vi "Power Enabled.vi"(0 "P CH":refnum<vi>, 1 "P CH_char":refnum<vi>, 2 "P CH, V":refnum<vi>, 3 "P CH_curlim, A":refnum<vi>, 4 "P CH_cur, A":refnum<vi>, 5 "P CH_selcur, A":refnum<vi>, 6 "P CH_counter":refnum<vi>, 7 "P CH_warning":refnum<vi>, 10 "P CH Used":bool, 16 "Stop":bool) -> ()   [LabVIEW 2018]
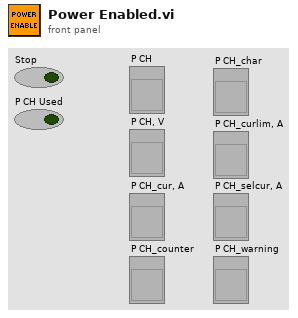
[diagram p1: front panel]
types:
  T1 = enum8{"Enabled", "Disabled", "Disabled and Grayed Out"}
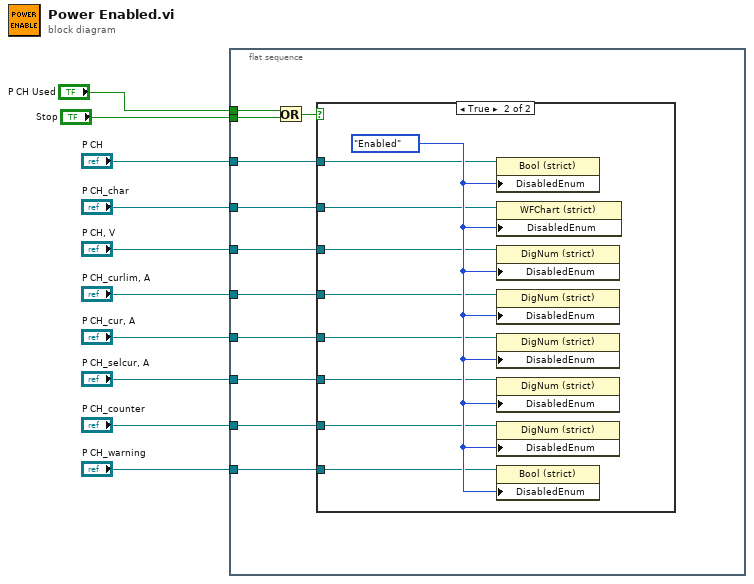
[diagram p0: block diagram]
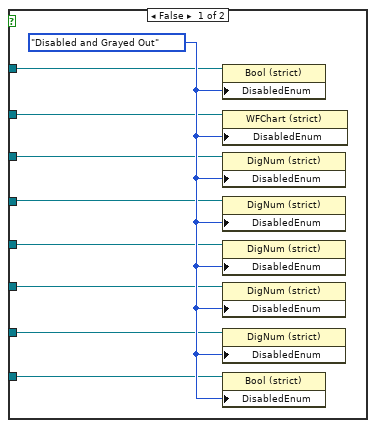
[diagram p2: hidden frame]
diagram:
  n1 = flat-sequence {
    tunnel: "Stop" -> [w20]
    tunnel: "P CH Used" -> [w19]
    tunnel: "P CH" -> [w18]
    tunnel: "P CH_char" -> [w17]
    tunnel: "P CH, V" -> [w16]
    tunnel: "P CH_curlim, A" -> [w15]
    tunnel: "P CH_cur, A" -> [w14]
    tunnel: "P CH_selcur, A" -> [w13]
    tunnel: "P CH_counter" -> [w12]
    tunnel: "P CH_warning" -> [w11]
    frame #0 {
      n2 = Or(x=w19, y=w20) -> (x .or. y?=w21:bool)
      n3 = case shown="True" w21 {
        tunnel: w18 -> [w29 w38]
        tunnel: w17 -> [w28 w37]
        tunnel: w16 -> [w27 w36]
        tunnel: w15 -> [w26 w35]
        tunnel: w14 -> [w25 w34]
        tunnel: w13 -> [w24 w33]
        tunnel: w12 -> [w23 w32]
        tunnel: w11 -> [w22 w31]
        frame False {
          w30 = T1."Disabled and Grayed Out" ("Disabled")
          n4 = property on="Property Node" class="Bool (strict)"(reference=w29, "DisabledEnum"=w30) -> ()  [unwired: 1 in, 2 out]
          n5 = property on="Property Node" class="WFChart (strict)"(reference=w28, "DisabledEnum"=w30) -> ()  [unwired: 1 in, 2 out]
          n6 = property on="Property Node" class="DigNum (strict)"(reference=w27, "DisabledEnum"=w30) -> ()  [unwired: 1 in, 2 out]
          n7 = property on="Property Node" class="DigNum (strict)"(reference=w26, "DisabledEnum"=w30) -> ()  [unwired: 1 in, 2 out]
          n8 = property on="Property Node" class="DigNum (strict)"(reference=w25, "DisabledEnum"=w30) -> ()  [unwired: 1 in, 2 out]
          n9 = property on="Property Node" class="DigNum (strict)"(reference=w24, "DisabledEnum"=w30) -> ()  [unwired: 1 in, 2 out]
          n10 = property on="Property Node" class="DigNum (strict)"(reference=w23, "DisabledEnum"=w30) -> ()  [unwired: 1 in, 2 out]
          n11 = property on="Property Node" class="Bool (strict)"(reference=w22, "DisabledEnum"=w30) -> ()  [unwired: 1 in, 2 out]
        }
        frame True {
          w39 = T1."Enabled" ("Disabled")
          n12 = property on="Property Node" class="Bool (strict)"(reference=w38, "DisabledEnum"=w39) -> ()  [unwired: 1 in, 2 out]
          n13 = property on="Property Node" class="WFChart (strict)"(reference=w37, "DisabledEnum"=w39) -> ()  [unwired: 1 in, 2 out]
          n14 = property on="Property Node" class="DigNum (strict)"(reference=w36, "DisabledEnum"=w39) -> ()  [unwired: 1 in, 2 out]
          n15 = property on="Property Node" class="DigNum (strict)"(reference=w35, "DisabledEnum"=w39) -> ()  [unwired: 1 in, 2 out]
          n16 = property on="Property Node" class="DigNum (strict)"(reference=w34, "DisabledEnum"=w39) -> ()  [unwired: 1 in, 2 out]
          n17 = property on="Property Node" class="DigNum (strict)"(reference=w33, "DisabledEnum"=w39) -> ()  [unwired: 1 in, 2 out]
          n18 = property on="Property Node" class="DigNum (strict)"(reference=w32, "DisabledEnum"=w39) -> ()  [unwired: 1 in, 2 out]
          n19 = property on="Property Node" class="Bool (strict)"(reference=w31, "DisabledEnum"=w39) -> ()  [unwired: 1 in, 2 out]
        }
      }
    }
  }
